vi "Example - Screwdriver Engage.vi"() -> ()   [LabVIEW 2017]
uses:
  SmartMotor_class/utils/SmartMotor Error.ctl
  SmartMotor_class/SmartMotor.lvclass
panel:
  in  "SmartMotor Chain Address":i16=1 min=1 max=10 step=1
  out "Screw Engaged":bool
  in  "Number of Tries":i32=1
  in  "Quit Program":bool
  in  "Engage":bool
  out "Error Out":errorcluster
  out "SmartMotor Error":T1
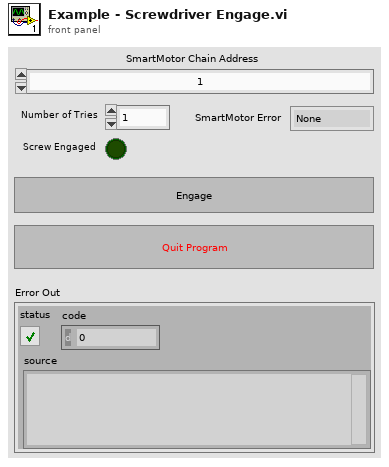
[diagram p1: front panel]
types:
  T1 = typedef "SmartMotor.lvclass/SmartMotor Error.ctl" = enum8{"None", "Read Error", "Low Voltage"}
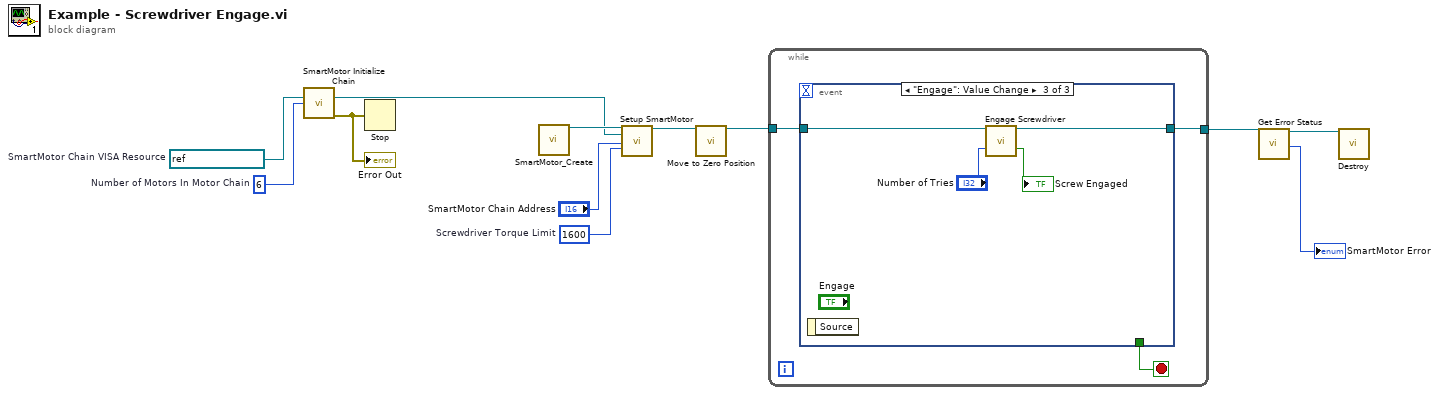
[diagram p0: block diagram]
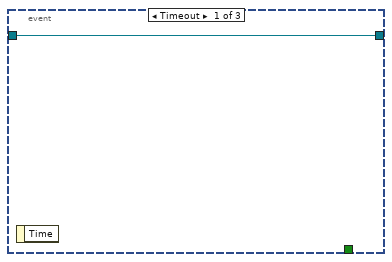
[diagram p2: hidden frame]
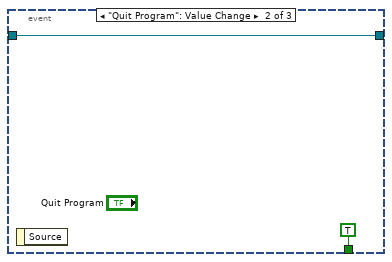
[diagram p3: hidden frame]
diagram:
  w3 = 6  # Number of Motors In Motor Chain
  w4 = refnum<visa-resource-name> "Serial-Hub-1"  # SmartMotor Chain VISA Resource
  w11 = 1600  # Screwdriver Torque Limit
  n1 = call "SmartMotor Initialize Chain.vi"("SmartMotor Chain VISA Resource"=w4, "Number of Motors In Motor Chain"=w3) -> ("SmartMotor Chain VISA Session"=w6:refnum<visa-resource-name>, "Error Out"=w5:errorcluster)  [unwired: 11 in, 1 out]
  "Error Out" <- w5
  n2 = Stop(stop? (T)=w5) -> ()
  n3 = call "SmartMotor_Create.vi"() -> ("reference out"=w12:refnum<class "SmartMotor.lvclass">)  [unwired: 18 in, 1 out]
  n4 = call-dynamic "Setup SmartMotor.vi"("reference in"=w12, "SmartMotor Chain VISA Session"=w6, "SmartMotor Chain Address"="SmartMotor Chain Address", "Screwdriver Torque Limit"=w11) -> ("reference out"=w10:refnum<class "SmartMotor.lvclass">)  [unwired: 13 in, 2 out]
  n5 = call-dynamic "Move to Zero Position.vi"("reference in"=w10) -> ("reference out"=w2:refnum<class "SmartMotor.lvclass">)  [unwired: 17 in, 1 out]
  n6 = while {
    tunnel: w2 -> [w15]
    tunnel: [w14] -> w8
    stop <- w13 stop-if-true
    n7 = event shown="[2] \"Engage\": Value Change" {
      selector: _ -> [_ _ _]
      dyn-events: _ -> [_ _ _]
      timeout: _ -> [_ _ _]
      tunnel: w15 -> [w16 w18 w19]
      tunnel: [w16 w18 w20] -> w14
      tunnel: [_ TRUE ("Quit Program") _] -> w13
      event Timeout {
        n8 = event-data() -> ()  [unwired: 1 in, 1 out]
      }
      event "Quit Program": Value Change {
        n9 = event-data() -> ()  [unwired: 1 in, 1 out]
      }
      event "Engage": Value Change {
        n10 = event-data() -> ()  [unwired: 1 in, 1 out]
        n11 = call-dynamic "Engage Screwdriver.vi"("reference in"=w19, "Number of Tries"="Number of Tries") -> ("reference out"=w20:refnum<class "SmartMotor.lvclass">, "Screw Engaged"=→"Screw Engaged":bool)  [unwired: 15 in, 1 out]
      }
    }
  }
  n12 = call-dynamic "Get Error Status.vi"("reference in"=w8) -> ("reference out"=w9:refnum<class "SmartMotor.lvclass">, "SmartMotor Error"=→"SmartMotor Error":T1)  [unwired: 16 in, 1 out]
  n13 = call-dynamic "Destroy.vi"("reference in"=w9) -> ()  [unwired: 17 in, 2 out]
